vi "Read RGB.vi"(8 "错误输入（无错误）":errorcluster, 9 "Pulse OUT":u8, 10 "S0S1S2S3":u8[](array[numeric]), 11 "LINX Resource输入":T1) -> (0 "错误输出":errorcluster, 1 "Blue":dbl, 2 "Green":dbl, 3 "Red":dbl, 5 "LINX Resource输出":T1)   [LabVIEW 2017]
uses:
  <vilib>/MakerHub/LINX/Private/Type Defs/LINX Ref.ctl
  <vilib>/MakerHub/LINX/Private/Type Defs/Platform.ctl
  <vilib>/MakerHub/LINX/Private/Type Defs/Interface.ctl
  <vilib>/MakerHub/LINX/Private/Device/Type Defs/LINX Device Config.ctl
  <vilib>/MakerHub/LINX/Private/Device/Type Defs/TCP Config.ctl
  <vilib>/MakerHub/LINX/Private/Device/Type Defs/Channels.ctl
  <vilib>/MakerHub/LINX/Public/Peripherals/Digital/Digital Write N Chans.vi
  <vilib>/MakerHub/LINX/Private/Local IO/LinxDigitalWrite.vi
  <vilib>/MakerHub/LINX/Public/Utilities/Check Channel.vi
  <vilib>/MakerHub/LINX/Private/Utilties/Generate Error.vi
  <vilib>/MakerHub/LINX/LMH-LINX.lvlib
  <vilib>/MakerHub/LINX/Private/Device/Device.lvlib
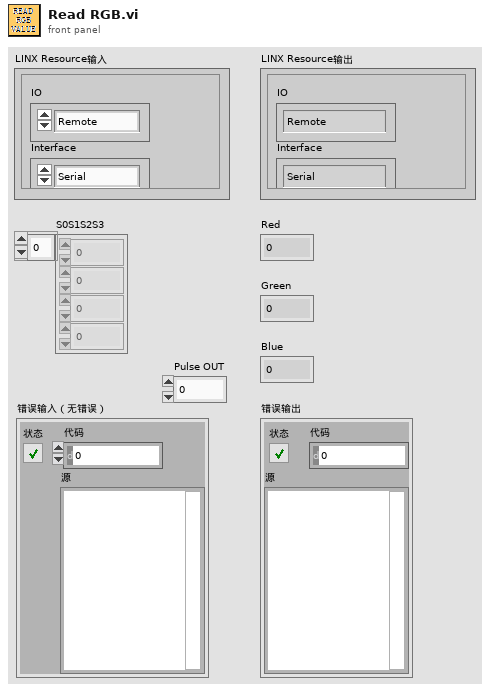
[diagram p1: front panel]
types:
  T1 = typedef "LMH-LINX.lvlib/LINX Ref.ctl" = cluster{"IO":T2, "Interface":T3, "LINX Device Config":T4}
  T2 = typedef "LMH-LINX.lvlib/Platform.ctl" = enum16{"Remote", "Local"}
  T3 = typedef "LMH-LINX.lvlib/Interface.ctl" = enum16{"Serial", "TCP"}
  T4 = typedef "LMH-LINX.lvlib/Device.lvlib/LINX Device Config.ctl" = cluster{"Interface":T3, "COM Port":refnum<visa-resource-name>, "TCP Configuration":T5, "Device Family":u8, "Device ID":u8, "Device Name":string, "TCP Ref":refnum<k5>, "Channels":T6}
  T5 = typedef "LMH-LINX.lvlib/Device.lvlib/TCP Config.ctl" = cluster{"IP Address":string, "Port":u16}
  T6 = typedef "LMH-LINX.lvlib/Channels.ctl" = cluster{"DI":u8[], "DO":u8[], "AI":u8[], "AO":u8[], "PWM":u8[], "QE":u8[], "UART":u8[], "I2C 2":u8[], "SPI":u8[], "CAN":u8[], "Servo":u8[], "AI Ref (V)":dbl, "AI Resolution (Bits)":u8, "AO Ref (V)":dbl, "AO Resolution (Bits)":u8}
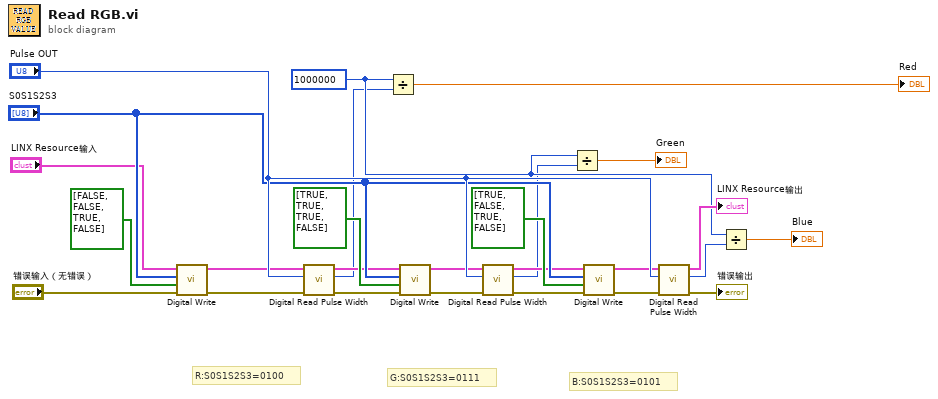
[diagram p0: block diagram]
diagram:
  w21 = u32 1000000 ("x")
  # "B:S0S1S2S3=0101"
  # "G:S0S1S2S3=0111"
  # "R:S0S1S2S3=0100"
  n1 = call-poly <vilib>:"Digital Write.vi"("Error In"="错误输入（无错误）", "Values"=bool[] [FALSE, FALSE, TRUE, FALSE], "DO Channels"="S0S1S2S3", "LINX Resource"="LINX Resource输入") -> ("Error Out"=w5:errorcluster, "LINX Resource"=w4:T1)  [unwired: 6 in]
  n2 = call <vilib>:"Digital Read Pulse Width.vi"("Error In"=w5, "DI Channel"="Pulse OUT", "LINX Resource"=w4) -> ("Error Out"=w9:errorcluster, "Pulse Width (uS)"=w7:u32, "LINX Resource"=w8:T1)  [unwired: 6 in]
  n3 = Divide(x=w21, y=w7) -> (x/y=→"Red":dbl)
  n4 = call-poly <vilib>:"Digital Write.vi"("Error In"=w9, "Values"=bool[] [TRUE, TRUE, TRUE, FALSE], "DO Channels"="S0S1S2S3", "LINX Resource"=w8) -> ("Error Out"=w12:errorcluster, "LINX Resource"=w11:T1)  [unwired: 6 in]
  n5 = call <vilib>:"Digital Read Pulse Width.vi"("Error In"=w12, "DI Channel"="Pulse OUT", "LINX Resource"=w11) -> ("Error Out"=w15:errorcluster, "Pulse Width (uS)"=w13:u32, "LINX Resource"=w14:T1)  [unwired: 6 in]
  n6 = Divide(x=w21, y=w13) -> (x/y=→"Green":dbl)
  n7 = call-poly <vilib>:"Digital Write.vi"("Error In"=w15, "Values"=bool[] [TRUE, FALSE, TRUE, FALSE], "DO Channels"="S0S1S2S3", "LINX Resource"=w14) -> ("Error Out"=w19:errorcluster, "LINX Resource"=w18:T1)  [unwired: 6 in]
  n8 = call <vilib>:"Digital Read Pulse Width.vi"("Error In"=w19, "DI Channel"="Pulse OUT", "LINX Resource"=w18) -> ("Error Out"=→"错误输出":errorcluster, "Pulse Width (uS)"=w22:u32, "LINX Resource"=→"LINX Resource输出":T1)  [unwired: 6 in]
  n9 = Divide(x=w21, y=w22) -> (x/y=→"Blue":dbl)
